vi "bol_tdms_write.vi"(7 "Boolean Data in":bool[][](array[boolean]), 8 "error in (no error)":errorcluster, 9 "channel name(s) in":string[](array[string]), 10 "Subsystem name in":string, 11 "tdms file":refnum<k34>) -> (0 "error out":errorcluster, 2 "Subsystem name out":string, 3 "tdms file out":refnum<k34>)   [LabVIEW 2017, in "labview-standard-library.lvlib" / "data-logging.lvlib"]
uses:
  data-logging.lvlib
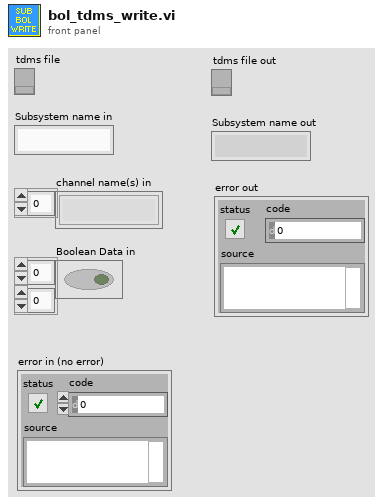
[diagram p1: front panel]
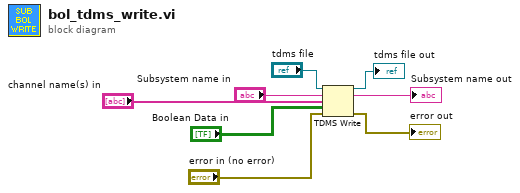
[diagram p0: block diagram]
diagram:
  n1 = TDMS Write(0:"tdms file", 5:"Subsystem name in", 7:"channel name(s) in", 9:"Boolean Data in", 11:"error in (no error)") -> (4:→"tdms file out":refnum<k34>, 6:→"Subsystem name out":string, 15:→"error out":errorcluster)  [unwired: 1 in, 1 out]
